vi "DriveConfigGlobal.vi"() -> ()   [LabVIEW 2022 SP3]
uses:
  DriveProperties.ctl
  Traverse Type.ctl
panel:
  in  "Channel Properties":T1[](array[typedef]) {"Current Pos" format="%.2f"; "Backlash/Eng units" format="%.2f"; "Pulses/rev" format="%.2f"; "Pos Tolerance" format="%.2f"; "Pulses/unit" format="%.2f"; "Acc. Min" format="%.2f"; "Acc. Max" format="%.2f"; "Vel. Min" format="%.2f"; "Vel. Max" format="%.2f"; "Acc. Default" format="%.2f"; "Vel. Default" format="%.2f"}
  in  "Stop Pressed?":bool
  in  "Run Emergency stop loop":bool
  in  "Position Offset XYZ":dbl[](array[numeric])=[0.0, 0.0, 0.0] format="%.2f"
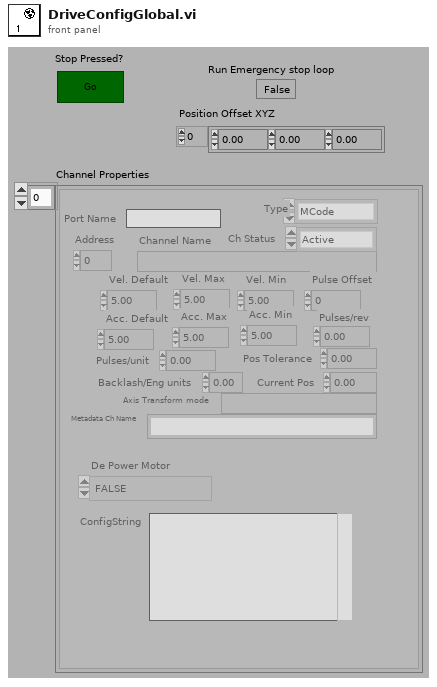
[diagram p1: front panel]
types:
  T1 = typedef "DriveProperties.ctl" = cluster{"Channel Name":string, "Vel. Default":sgl, "Acc. Default":sgl, "Vel. Max":sgl, "Vel. Min":sgl, "Acc. Max":sgl, "Acc. Min":sgl, "Pulses/unit":sgl, "Address":u8, "Pulse Offset":i32, "Pos Tolerance":sgl, "Pulses/rev":sgl, "Backlash/Eng units":sgl, "Current Pos":sgl, "Ch Status":enum16{"Active", "Offline", "Simulate"}, "Port Name":string, "Axis Transform mode":string, "Metadata Ch Name":string, "Type":T2, "De Power Motor":enum16{"TRUE", "FALSE"}, "ConfigString":string}
  T2 = typedef "Traverse Type.ctl" = enum16{"MCode", "Dynamixel"}
diagram:
